vi "Test_Multiple_Panel.vi"() -> ()   [LabVIEW 2021]
panel:
  out "Loading#":i32
  in  "Loading":bool
  in  "Exit":bool
  in  "Test Panel#":i32=5
  in  "Time Target (s)":dbl=5.0 format="%.0p"
  in  "System_Delay(s)":dbl=0.01 format="%.0p"
  in  "State_Interval_Time(s)":dbl=0.01 format="%.0p"
  in  "State#":i32=1000
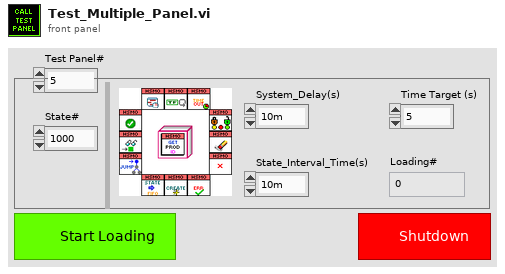
[diagram p1: front panel]
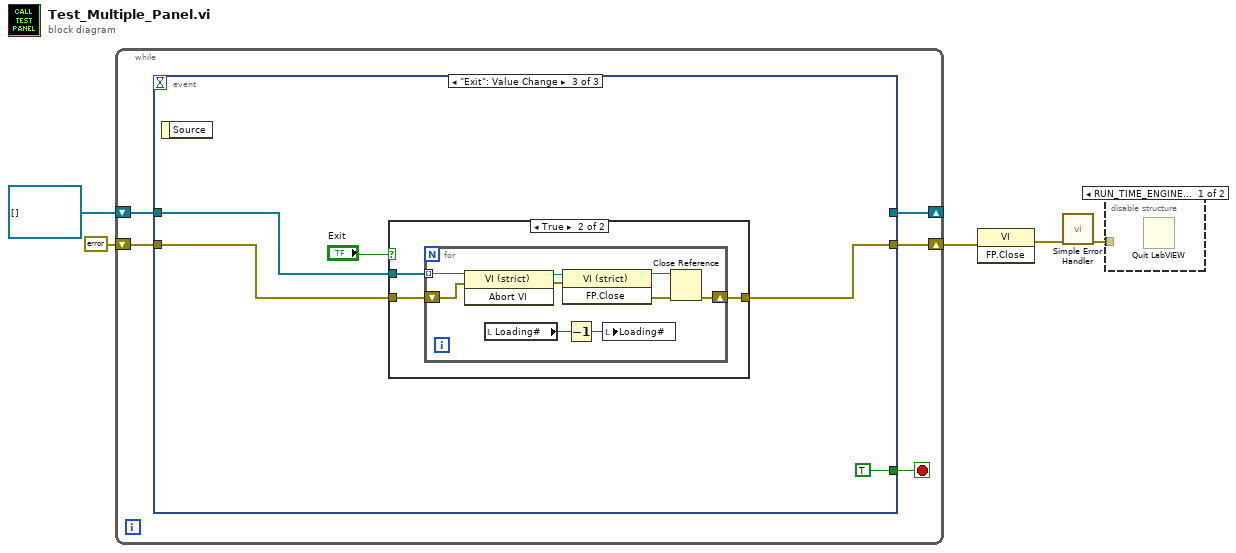
[diagram p0: block diagram]
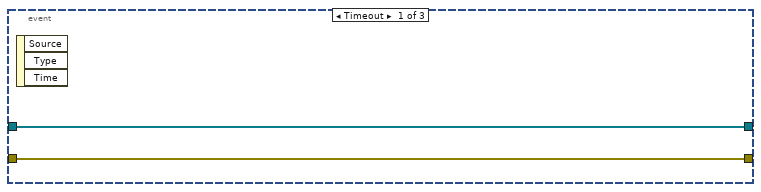
[diagram p3: hidden frame]
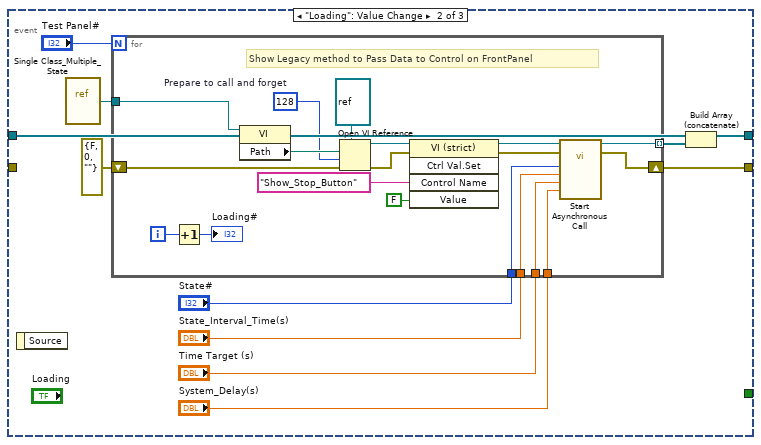
[diagram p4: hidden frame]
diagram:
  n1 = while {
    shift-right: [w10] -> _
    shift-left: refnum<vi>[] [] -> [w8]
    shift-right: [w9] -> w3
    shift-left: errorcluster {"status"=FALSE, "code"=0, "source"=""} ("error out") -> [w7]
    stop <- w6 stop-if-true
    n2 = event shown="[2] \"Exit\": Value Change" {
      selector: _ -> [_ _ _]
      dyn-events: _ -> [_ _ _]
      timeout: _ -> [_ _ _]
      tunnel: [w12 w14 _] -> w10
      tunnel: [w11 w15 w44] -> w9
      tunnel: w8 -> [w12 w13 w46]
      tunnel: w7 -> [w11 _ w45]
      tunnel: [_ _ TRUE] -> w6
      event Timeout {
        n3 = event-data() -> ()  [unwired: 1 in, 3 out]
      }
      event "Loading": Value Change {
        n4 = event-data() -> ()  [unwired: 1 in, 1 out]
        n5 = vi-ref "Single Class_Multiple_State.vi"() -> (w19:refnum<vi>)
        n6 = for {
          N: "Test Panel#" -> [_]
          shift-right: [w24] -> w15
          shift-left: errorcluster {"status"=FALSE, "code"=0, "source"=""} ("error out") -> [w26]
          tunnel: w19 -> [w40]
          tunnel: "State#" -> [w39]
          tunnel: "State_Interval_Time(s)" -> [w38]
          tunnel: "System_Delay(s)" -> [w37]
          tunnel: "Time Target (s)" -> [w36]
          tunnel: [w25] -> w16 mode=indexing
          i -> [w29]
          w35 = 128  # Prepare to call and forget
          # "Show Legacy method to Pass Data to Control on FrontPanel"
          n7 = Increment(x=w29) -> (x+1=→"Loading#":i32)
          n8 = property class="VI"(reference=w40) -> ("Path"=w42:path)  [unwired: 1 in, 2 out]
          n9 = Open VI Reference(type specifier VI Refnum (for type only)=refnum<vi> refnum, vi path=w42, options=w35, error in (no error)=w26) -> (vi reference=w27:refnum<vi>, error out=w32:errorcluster)  [unwired: 2 in]
          n10 = invoke class="VI (strict)" method="Ctrl Val.Set"(reference=w27, error in=w32, "Control Name"="Show_Stop_Button", "Value"=FALSE) -> (reference out=w33:refnum<vi>, error out=w34:errorcluster)  [unwired: 1 in, 3 out]
          n11 = call-by-ref "Start Asynchronous Call"(reference=w33, error in=w34, "System_Delay(s)"=w37, "Time Target (s)"=w36, "State_Interval_Time(s)"=w38, "State#"=w39) -> (reference out=w25:refnum<vi>, error out=w24:errorcluster)  [unwired: 4 in]
        }
        n12 = Build Array (concatenate)(w13, w16) -> (w14:refnum<vi>[])
      }
      event "Exit": Value Change {
        n13 = event-data() -> ()  [unwired: 1 in, 1 out]
        n14 = case shown="True" "Exit" {
          tunnel: w46 -> [_ w51]
          tunnel: w45 -> [w48 w50]
          tunnel: [w48 w49] -> w44
          frame False {
          }
          frame True {
            n15 = for {
              tunnel: w51 -> [w55] mode=indexing
              shift-right: [w56] -> w49
              shift-left: w50 -> [w52]
              n16 = invoke class="VI (strict)" method="Abort VI"(reference=w55, error in=w52) -> (reference out=w54:refnum<vi>, error out=w53:errorcluster)  [unwired: 1 in, 1 out]
              n17 = local read "Loading#"() -> (w58:i32)
              n18 = invoke class="VI (strict)" method="FP.Close"(reference=w54, error in=w53) -> (reference out=w60:refnum<vi>, error out=w59:errorcluster)  [unwired: 1 in, 1 out]
              n19 = Decrement(x=w58) -> (x-1=w57:i32)
              n20 = local write "Loading#"(w57) -> ()
              n21 = Close Reference(reference=w60, error in (no error)=w59) -> (error out=w56:errorcluster)
            }
          }
        }
      }
    }
  }
  n22 = invoke class="VI" method="FP.Close"(error in=w3) -> (error out=w5:errorcluster)  [unwired: 2 in, 2 out]
  n23 = call <vilib>:"Simple Error Handler.vi"("error in (no error)"=w5) -> ("error out"=w2:errorcluster)  [unwired: 4 in, 4 out]
  n24 = disable-structure shown="RUN_TIME_ENGINE==True" {
    disable-tunnel: w2 -> [_ _]
    frame condition #0 {
      n25 = Quit LabVIEW() -> ()  [unwired: 1 in]
    }
    frame condition #1 (active) {
    }
  }
